vi "Read RAW ADC.vi"(8 "error in (no error)":errorcluster, 10 "Channel":u32, 11 "VISA resource name":refnum<visa-resource-name>) -> (0 "error out":errorcluster, 2 "ADC Raw Value":u16 format="%.0x", 3 "VISA resource name out":refnum<visa-resource-name>)   [LabVIEW 2013, in "HadCon.lvlib"]
doc: "Read ADC raw value of specified channel."
uses:
  <instrlib>/HadCon/HadCon.lvlib
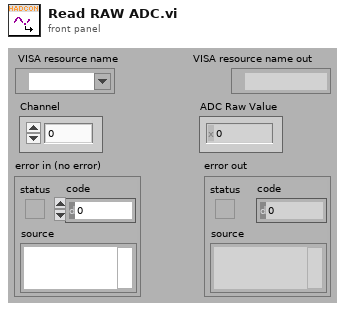
[diagram p1: front panel]
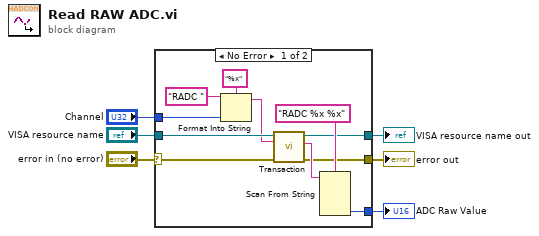
[diagram p0: block diagram]
diagram:
  n1 = case shown="No Error" "error in (no error)" {
    selector: "error in (no error)" -> [w13 w18]
    tunnel: [w8 w19] -> w6
    tunnel: "VISA resource name" -> [w17 w19]
    tunnel: [w7 w18] -> w4
    tunnel: "Channel" -> [w15 _]
    tunnel: [w10 _] -> w1
    frame No Error {
      n2 = Format Into String(format string="%x", initial string="RADC ", w15) -> (resulting string=w14:string)  [unwired: 1 in, 1 out]
      n3 = call <instrlib>:"Transaction.vi"("Error In"=w13, "Command"=w14, "VISA resource name"=w17) -> ("Error Out"=w7:errorcluster, "Response"=w12:string, "VISA resource name out"=w8:refnum<visa-resource-name>)  [unwired: 6 in]
      n4 = Scan From String(format string="RADC %x %x", input string=w12) -> (output 2=w10:u32)  [unwired: 5 in, 3 out]
    }
    frame Error {
    }
  }
  "VISA resource name out" <- w6
  "error out" <- w4
  "ADC Raw Value" <- w1
